vi "Stop Parse.vi"() -> ()   [LabVIEW 2025]
panel:
  in  "Stop Parse":bool
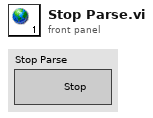
[diagram p1: front panel]
diagram:
